vi "Config Harmonics.vi"(0 "VISA resource name":refnum<visa-resource-name>, 1 "Element (1: Element 1)":u16(ring)=1 items=["", "Element1", "Element2", "Element3"], 5 "Harmonic Mode (F: OFF)":bool, 7 "PLL source (0: V1)":u16(ring) items=["V1", "A1", "V2", "A2", "V3", "A3"], 9 "THD (0: IEC)":u16(ring) items=["IEC", "CSA"], 11 "error in (no error)":errorcluster) -> (4 "VISA resource name out":refnum<visa-resource-name>, 15 "error out":errorcluster)   [LabVIEW 2016, in "Yokogawa WT200 Series.lvlib"]
doc: "This VI sends the Harmonics Configuration command to the WT200 Series.\n\nNote : It needs /HRM option."
uses:
  Yokogawa WT200 Series.lvlib
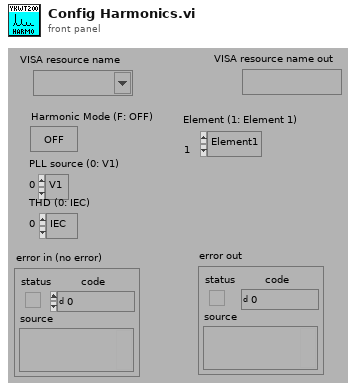
[diagram p1: front panel]
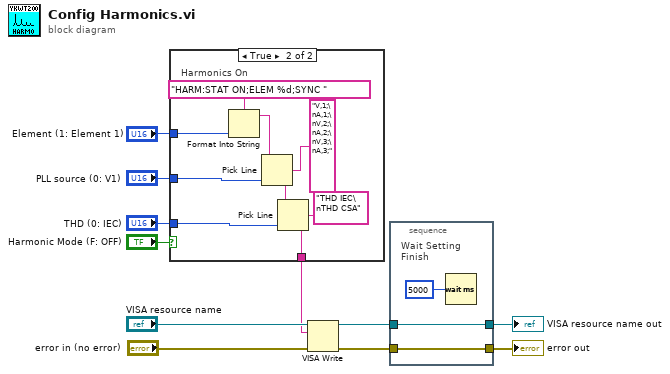
[diagram p0: block diagram]
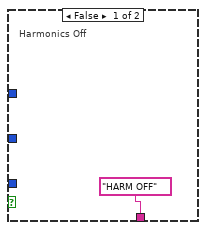
[diagram p2: hidden frame]
diagram:
  n1 = case shown="True" "Harmonic Mode (F: OFF)" {
    tunnel: "THD (0: IEC)" -> [_ w21]
    tunnel: ["HARM OFF" w19] -> w3
    tunnel: "PLL source (0: V1)" -> [_ w18]
    tunnel: "Element (1: Element 1)" -> [_ w14]
    frame False {
      # "Harmonics Off"
    }
    frame True {
      # "Harmonics On"
      n2 = Format Into String(format string="HARM:STAT ON;ELEM %d;SYNC ", w14) -> (resulting string=w15:string)  [unwired: 2 in, 1 out]
      n3 = Pick Line(string ("")=w15, multi-line string="V,1;\nA,1;\nV,2;\nA,2;\nV,3;\nA,3;", line index=w18) -> (output string=w16:string)
      n4 = Pick Line(string ("")=w16, multi-line string="THD IEC\nTHD CSA", line index=w21) -> (output string=w19:string)
    }
  }
  n5 = VISA Write(VISA resource name="VISA resource name", write buffer=w3, error in (no error)="error in (no error)") -> (VISA resource name out=w8:refnum<visa-resource-name>, error out=w9:errorcluster)  [unwired: 1 out]
  n6 = stacked-sequence {
    tunnel: w9 -> [w24]
    tunnel: [w24] -> w1
    tunnel: w8 -> [w23]
    tunnel: [w23] -> w7
    frame #0 {
      # "Wait Setting\nFinish"
      n7 = Wait (ms)(milliseconds to wait=u32 5000) -> ()  [unwired: 1 out]
    }
  }
  "VISA resource name out" <- w7
  "error out" <- w1
